vi "AppInit.vi"(10 "path":path, 11 "Changelog":string caption="App Ver") -> (0 "error out":errorcluster)   [LabVIEW 2016]
doc: "Init Host application"
uses:
  Tools/Windows/Windows.ExitAction.ctl
  Tools/EventLog/EventLog.Buffer.Action.ctl
  Tools/Translator/Translator.Message.ctl
  Tools/EventLog/EventLog.New(single).vi
  Global/ApplicationGlobal.vi
  Tools/Config/Config.Global.vi
  Tools/EventLog/EventLog.File.ReadWrite.vi
panel:
  out "idx":i32
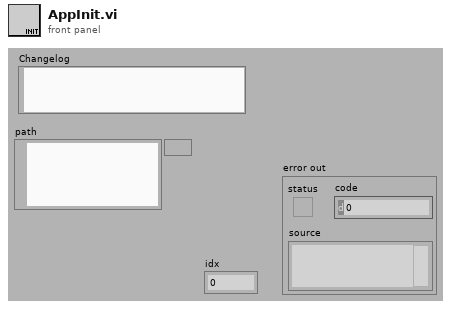
[diagram p1: front panel]
types:
  T1 = typedef "Windows.ExitAction.ctl" = enum16{"Log off from PC", "Shut Down PC", "Reboot PC", "Close Program"}
  T2 = typedef "EventLog.Buffer.Action.ctl" = enum16{"init", "re-init", "clear", "set translator", "translate", "add", "get"}
  T3 = typedef "Translator.Message.ctl" = enum16{"-", "Event confirmed", "Log out", "Log in", "Shutdown", "Cancel", "Start", "Continue", "Stop", "On", "Off", "OK", "NOK", "NOK %s", "This", "Prev", "Home", "Work", "In progress...", "Missing", "Empty", "Hardware failure", "Initial", "Error %d >> %s", "Error %d >> %s >> %s", "Starting %s", "Quitting %s", "Configured", "Initializing", "Quitting", "Loading", "Running %s", "Stopped", "Summary", "Do you want to continue?", "Do you want to exit?", "Log out?", "System", "All", "IDLE", "Translating...%s", "Not found", "Alarm %s", "Run", "Skip", "Abort", "Repeat", "Please wait...", "Database disconnected", "Login to database successful", "Login to database failed: %d; %s", "Get process step data for %s", "Changeover off", "Changeover into %s", "Product %s | %s found in cache with status %d at previous station", "Product %s | %s found in database with status %d at previous station", "Product %s | %s not found in cache at previous station", "Product %s | %s not found in database at previous station", "Product %s | %s found in cache with status %d at this station (%d repetion)", "Product %s | %s found in database with status %d at this station (%d repetition)", "Product %s | %s not found in cache at this station", "Product %s | %s not found in database at this station", "Product %s | %s found in cache for component %s | %s", "Product %s | %s found in database for component %s | %s", "Product not found in cache for component %s | %s", "Product not found in database for component %s | %s", "Product %s | %s connected with component %s | %s (cache)", "Product %s | %s connected with component %s | %s (database)", "New data for %s | %s (cache)", "New data for %s | %s (database)", "File %s moved (cache)", "File %s deleted (cache)", "Msg %d >> %s", "PLC LifeBit Failure", "Reconnecting DB", "Reconnecting PLC", "Free disk space is below 1GB - contact technician"}
  T4 = enum32{"invalid app kind", "Development System", "Run Time System", "Student Edition", "Embedded LabVIEW", "Evaluation", "Custom"}
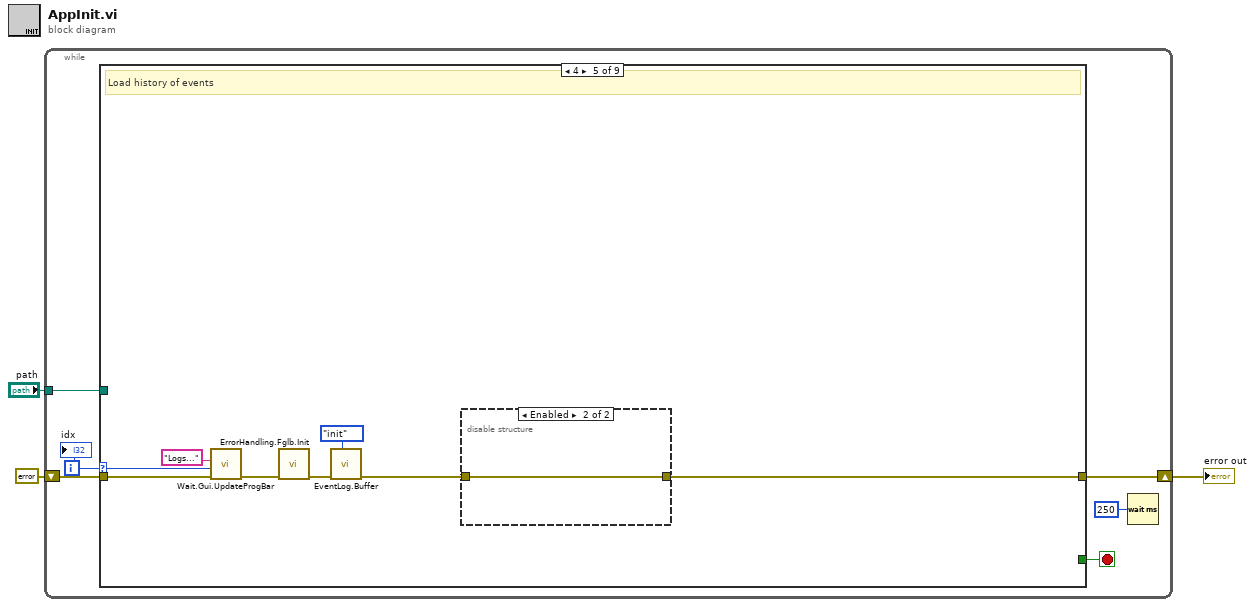
[diagram p0: block diagram]
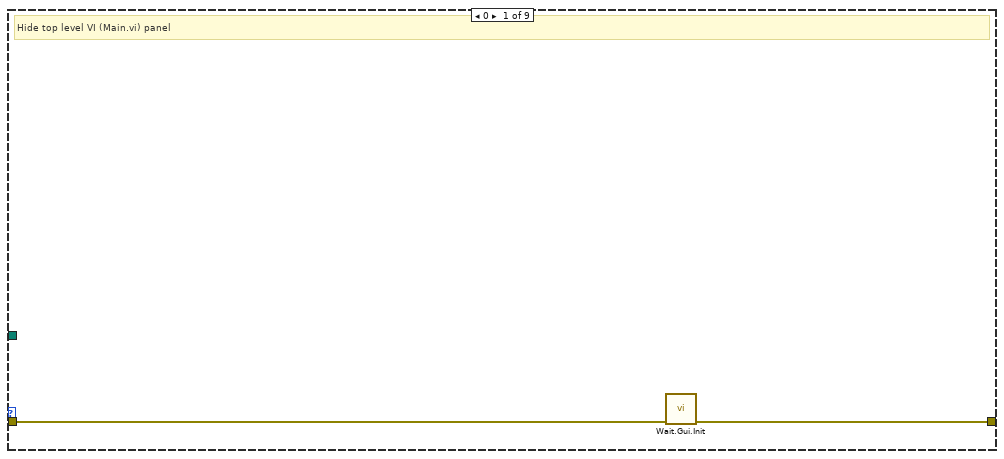
[diagram p2: hidden frame]
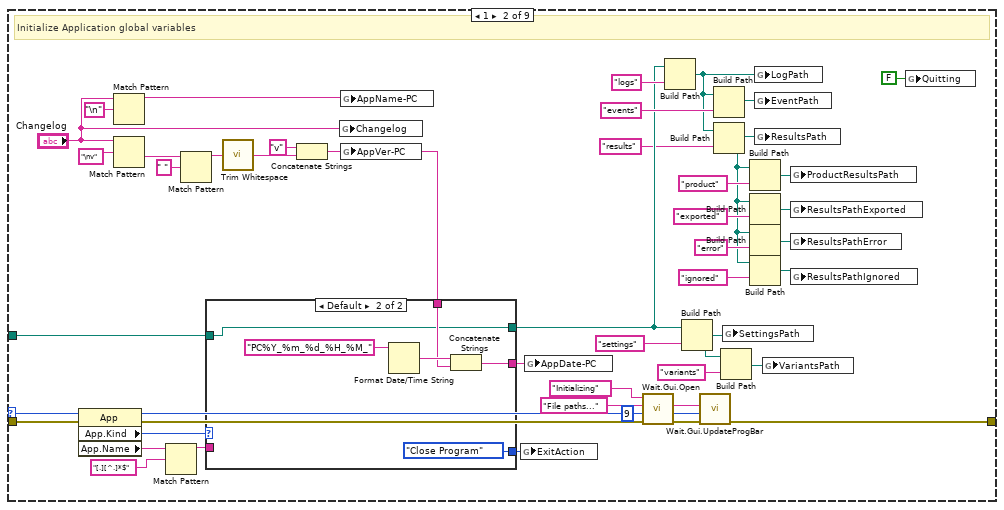
[diagram p3: hidden frame]
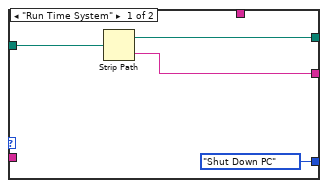
[diagram p4: hidden frame]
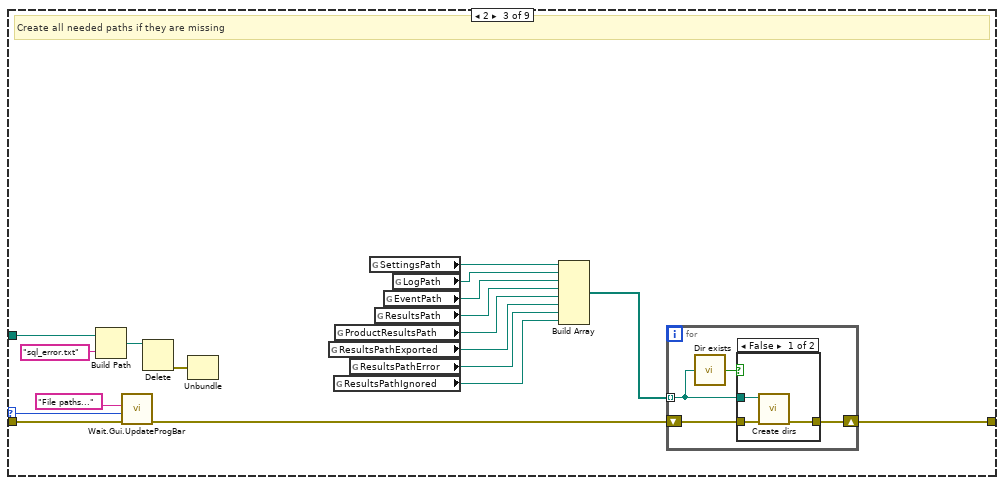
[diagram p5: hidden frame]
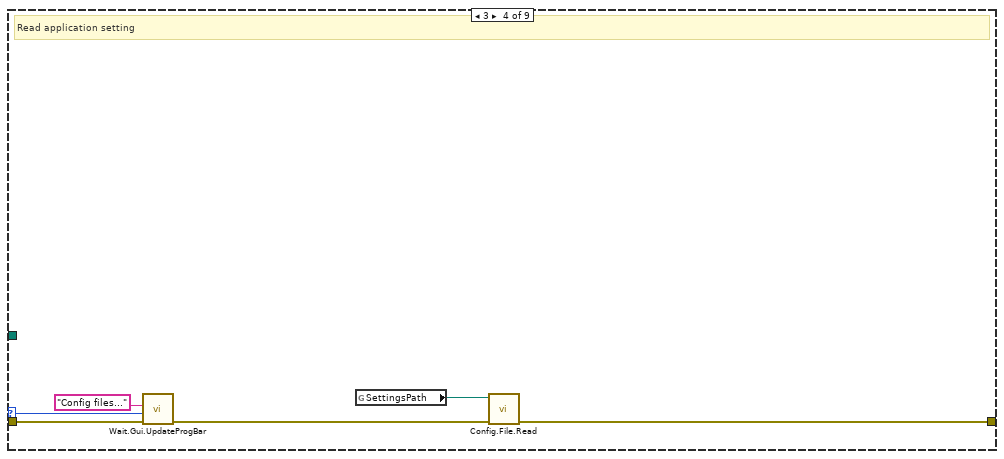
[diagram p7: hidden frame]
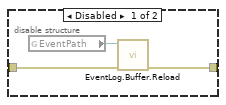
[diagram p8: hidden frame]
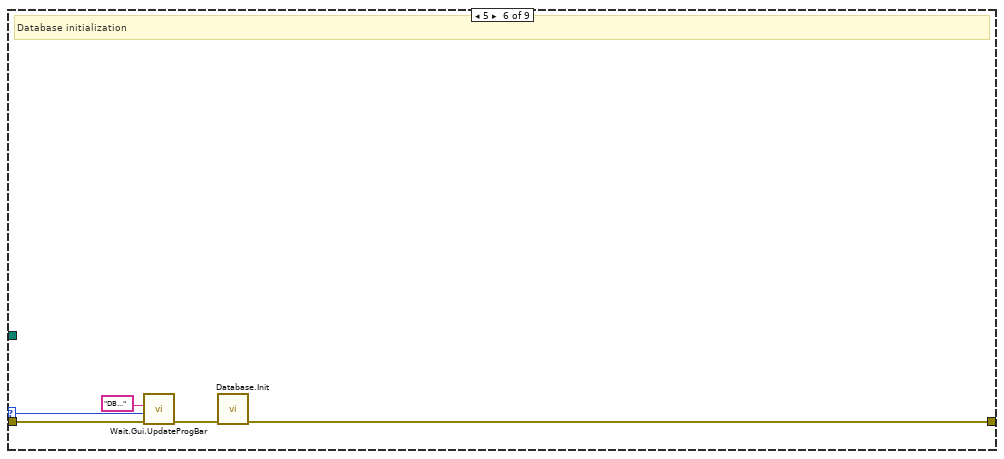
[diagram p9: hidden frame]
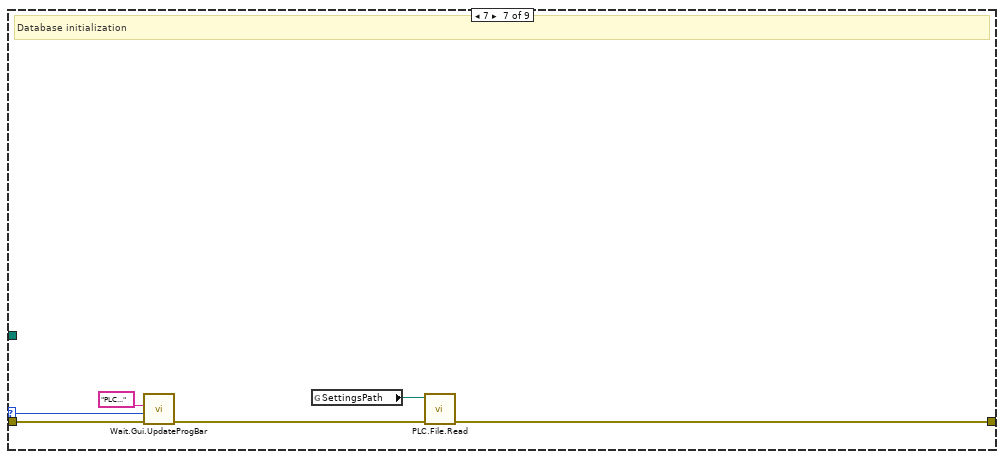
[diagram p10: hidden frame]
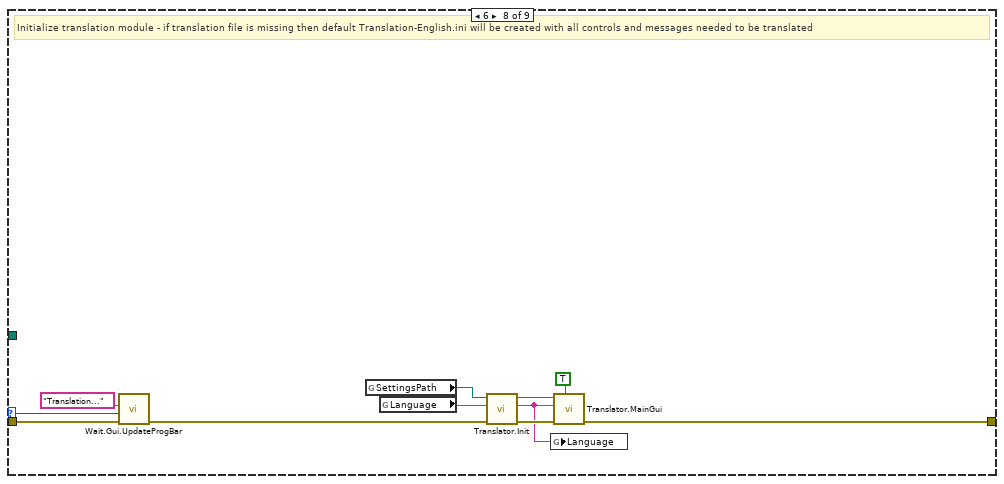
[diagram p11: hidden frame]
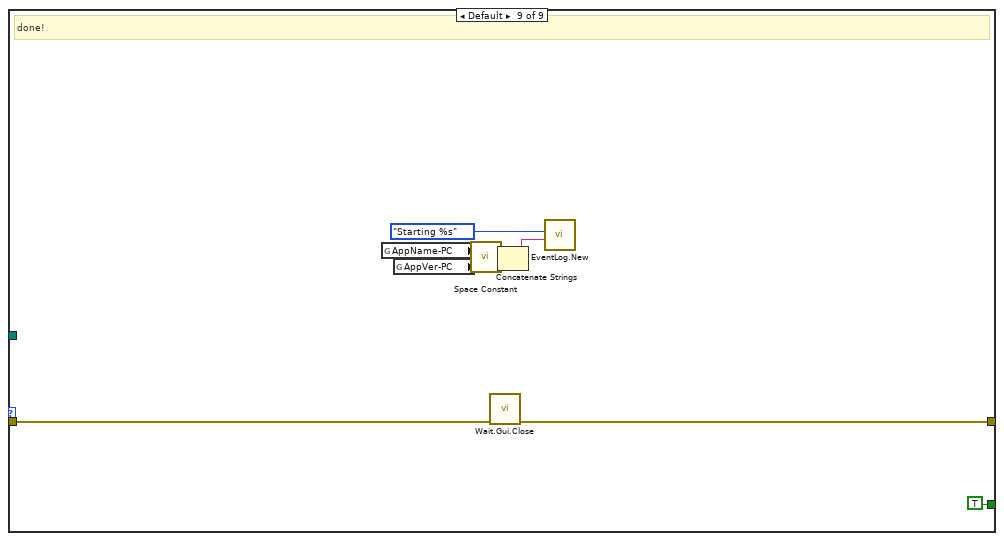
[diagram p12: hidden frame]
diagram:
  n1 = while {
    shift-right: [w7] -> w1
    shift-left: errorcluster {"status"=FALSE, "code"=0, "source"=""} ("error out") -> [w9]
    tunnel: "path" -> [w6]
    i -> [w5]
    stop <- w8 stop-if-true
    n2 = case shown="4" w5 {
      selector: w5 -> [_ w28 w78 w97 w102 w114 w121 w124 _]
      tunnel: w9 -> [w11 w46 w77 w96 w101 w113 w120 w125 w138]
      tunnel: [_ _ _ _ _ _ _ _ TRUE] -> w8
      tunnel: [w10 w29 w81 w93 w99 w115 w117 w123 w137] -> w7
      tunnel: w6 -> [_ w37 w73 _ _ _ _ _ _]
      frame 0 {
        # "Hide top level VI (Main.vi) panel"
        n3 = call "Wait.Gui.Init.vi"("error in (no error)"=w11) -> ("error out"=w10:errorcluster)  [unwired: 10 in]
      }
      frame 1 {
        w32 = "File paths..."
        # "Initialize Application global variables"
        n4 = property class="App"(error in=w46) -> (error out=w30:errorcluster, "App.Kind"=w47:T4, "App.Name"=w40:string)  [unwired: 1 in, 1 out]
        n5 = Match Pattern(string="Changelog", regular expression="\n") -> (before substring=w35:string)  [unwired: 1 in, 3 out]
        n6 = Match Pattern(string="Changelog", regular expression="\nv") -> (after substring=w54:string)  [unwired: 1 in, 3 out]
        n7 = Match Pattern(string=w40, regular expression="[.][^.]*$") -> (before substring=w39:string)  [unwired: 4 out]
        n8 = Match Pattern(string=w54, regular expression=" ") -> (before substring=w51:string)  [unwired: 1 in, 3 out]
        n9 = call <vilib>:"Trim Whitespace.vi"("string"=w51) -> ("trimmed string"=w49:string)  [unwired: 1 in]
        n10 = Concatenate Strings("v" ("string"), w49) -> (w34:string)
        n11 = case shown="Default" w47 {
          tunnel: [w58 w64] -> w43
          tunnel: w34 -> [_ w63]
          tunnel: [w60 w62] -> w27
          tunnel: w39 -> [_ _]
          tunnel: w37 -> [w59 w62]
          tunnel: [Windows.ExitAction."Shut Down PC" ("ExitAction") Windows.ExitAction."Close Program" ("ExitAction")] -> w26
          frame "Run Time System" {
            n12 = Strip Path(path=w59) -> (stripped path=w60:path, name=w58:string)
          }
          frame Default {
            n13 = Format Date/Time String(time format string (%c)="PC%Y_%m_%d_%H_%M_") -> (date/time string=w65:string)  [unwired: 2 in]
            n14 = Concatenate Strings(w65, w63) -> (w64:string)
          }
        }
        n15 = global write "ApplicationGlobal.vi" "Changelog"("Changelog") -> ()
        n16 = global write "ApplicationGlobal.vi" "AppName-PC"(w35) -> ()
        n17 = global write "ApplicationGlobal.vi" "AppVer-PC"(w34) -> ()
        n18 = global write "ApplicationGlobal.vi" "ExitAction"(w26) -> ()
        n19 = global write "ApplicationGlobal.vi" "AppDate-PC"(w43) -> ()
        n20 = call "Wait.Gui.Open.vi"("error in (no error)"=w30, "ProgBarSize (0)"=9 ("ProgBarSize"), "Status (\"\")"=w32, "Msg"="Initializing" ("format string")) -> ("error out"=w33:errorcluster)  [unwired: 7 in]
        n21 = Build Path(base path=w27, name or relative path="logs") -> (appended path=w21:path)
        n22 = Build Path(base path=w27, name or relative path="settings") -> (appended path=w23:path)
        n23 = call "Wait.Gui.UpdateProgBar.vi"("error in (no error)"=w33, "ProgBar (0)"=w28, "status (\"\")"=w32) -> ("error out"=w29:errorcluster)  [unwired: 8 in]
        n24 = Build Path(base path=w21, name or relative path="events") -> (appended path=w42:path)
        n25 = Build Path(base path=w21, name or relative path="results") -> (appended path=w15:path)
        n26 = Build Path(base path=w23, name or relative path="variants") -> (appended path=w22:path)
        n27 = global write "ApplicationGlobal.vi" "SettingsPath"(w23) -> ()
        n28 = Build Path(base path=w15, name or relative path="product") -> (appended path=w19:path)
        n29 = Build Path(base path=w15, name or relative path="exported") -> (appended path=w14:path)
        n30 = Build Path(base path=w15, name or relative path="error") -> (appended path=w13:path)
        n31 = Build Path(base path=w15, name or relative path="ignored") -> (appended path=w12:path)
        n32 = global write "ApplicationGlobal.vi" "LogPath"(w21) -> ()
        n33 = global write "ApplicationGlobal.vi" "EventPath"(w42) -> ()
        n34 = global write "ApplicationGlobal.vi" "ResultsPath"(w15) -> ()
        n35 = global write "ApplicationGlobal.vi" "VariantsPath"(w22) -> ()
        n36 = global write "ApplicationGlobal.vi" "ProductResultsPath"(w19) -> ()
        n37 = global write "ApplicationGlobal.vi" "ResultsPathExported"(w14) -> ()
        n38 = global write "ApplicationGlobal.vi" "ResultsPathError"(w13) -> ()
        n39 = global write "ApplicationGlobal.vi" "ResultsPathIgnored"(w12) -> ()
        n40 = global write "ApplicationGlobal.vi" "Quitting"(FALSE ("Quitting")) -> ()
      }
      frame 2 {
        # "Create all needed paths if they are missing"
        n41 = Build Path(base path=w73, name or relative path="sql_error.txt") -> (appended path=w74:path)
        n42 = call "Wait.Gui.UpdateProgBar.vi"("error in (no error)"=w77, "ProgBar (0)"=w78, "status (\"\")"="File paths...") -> ("error out"=w76:errorcluster)  [unwired: 8 in]
        n43 = Delete(path (use dialog)=w74) -> (error out=w72:errorcluster)  [unwired: 4 in, 2 out]
        n44 = Unbundle(w72) -> ()  [unwired: 3 out]
        n45 = global read "ApplicationGlobal.vi" "ResultsPathExported"() -> (w69:path)
        n46 = global read "ApplicationGlobal.vi" "ResultsPathIgnored"() -> (w67:path)
        n47 = global read "ApplicationGlobal.vi" "ProductResultsPath"() -> (w71:path)
        n48 = global read "ApplicationGlobal.vi" "ResultsPathError"() -> (w68:path)
        n49 = global read "ApplicationGlobal.vi" "SettingsPath"() -> (w84:path)
        n50 = global read "ApplicationGlobal.vi" "ResultsPath"() -> (w70:path)
        n51 = global read "ApplicationGlobal.vi" "EventPath"() -> (w82:path)
        n52 = global read "ApplicationGlobal.vi" "LogPath"() -> (w83:path)
        n53 = Build Array(w84, w83, w82, w70, w71, w69, w68, w67) -> (w80:path[])
        n54 = for {
          tunnel: w80 -> [w86] mode=indexing
          shift-right: [w87] -> w81
          shift-left: w76 -> [w88]
          n55 = call "Dir exists.vi"("dir path"=w86) -> ("exists?"=w85:bool)  [unwired: 4 in]
          n56 = case shown="False" w85 {
            tunnel: w86 -> [w91 _]
            tunnel: w88 -> [w90 w92]
            tunnel: [w89 w92] -> w87
            frame False {
              n57 = call "Create dirs.vi"("error in (no error)"=w90, "deepest dir"=w91) -> ("error"=w89:errorcluster)  [unwired: 9 in]
            }
            frame True {
            }
          }
        }
      }
      frame 3 {
        # "Read application setting"
        n58 = call "Wait.Gui.UpdateProgBar.vi"("error in (no error)"=w96, "ProgBar (0)"=w97, "status (\"\")"="Config files...") -> ("error out"=w94:errorcluster)  [unwired: 8 in]
        n59 = global read "ApplicationGlobal.vi" "SettingsPath"() -> (w95:path)
        n60 = call "Config.File.Read.vi"("error in"=w94, "path"=w95) -> ("error out"=w93:errorcluster)  [unwired: 9 in]
      }
      frame 4 {
        # "Load history of events"
        n61 = call "Wait.Gui.UpdateProgBar.vi"("error in (no error)"=w101, "ProgBar (0)"=w102, "status (\"\")"="Logs...") -> ("error out"=w100:errorcluster)  [unwired: 8 in]
        n62 = call "ErrorHandling.Fglb.Init.vi"("error in (no error)"=w100) -> ("error out"=w104:errorcluster)  [unwired: 10 in]
        n63 = call "EventLog.Buffer.vi"("action (get)"=EventLog.Buffer.Action."init" ("action (read)"), "error in"=w104) -> ("error out"=w105:errorcluster)  [unwired: 6 in, 3 out]
        n64 = disable-structure shown="Enabled" {
          disable-tunnel: [w108 w110] -> w99
          disable-tunnel: w105 -> [w107 w110]
          frame Disabled {
            n65 = global read "ApplicationGlobal.vi" "EventPath"() -> (w109:path)
            n66 = call "EventLog.Buffer.Reload.vi"("error in"=w107, "Path"=w109) -> ("error out"=w108:errorcluster)  [unwired: 9 in]
          }
          frame Enabled {
          }
        }
      }
      frame 5 {
        # "Database initialization"
        n67 = call "Wait.Gui.UpdateProgBar.vi"("error in (no error)"=w113, "ProgBar (0)"=w114, "status (\"\")"="DB...") -> ("error out"=w111:errorcluster)  [unwired: 8 in]
        n68 = call "Database.Init.vi"("error in (no error)"=w111) -> ("error out"=w115:errorcluster)  [unwired: 10 in]
      }
      frame 7 {
        # "Database initialization"
        n69 = call "Wait.Gui.UpdateProgBar.vi"("error in (no error)"=w120, "ProgBar (0)"=w121, "status (\"\")"="PLC...") -> ("error out"=w118:errorcluster)  [unwired: 8 in]
        n70 = global read "ApplicationGlobal.vi" "SettingsPath"() -> (w116:path)
        n71 = call "PLC.File.Read.vi"("error in"=w118, "path"=w116) -> ("error out"=w117:errorcluster)  [unwired: 9 in]
      }
      frame 6 {
        # "Initialize translation module - if translation file is missing then default Translation-English.ini will be created with all controls and messages needed to be translated"
        n72 = call "Wait.Gui.UpdateProgBar.vi"("error in (no error)"=w125, "ProgBar (0)"=w124, "status (\"\")"="Translation...") -> ("error out"=w122:errorcluster)  [unwired: 8 in]
        n73 = global read "ApplicationGlobal.vi" "SettingsPath"() -> (w129:path)
        n74 = global read "Config.Global.vi" "Language"() -> (w130:string)
        n75 = call "Translator.Init.vi"("error in"=w122, "Language in"=w130, "Translation folder"=w129) -> ("error out"=w131:errorcluster, "Language out"=w128:string)  [unwired: 7 in]
        n76 = global write "Config.Global.vi" "Language"(w128) -> ()
        n77 = call "Translator.MainGui.vi"("~init (F)"=TRUE ("init (F)"), "~error in"=w131, "~Language in use"=w128, "~Translation folder"=w129) -> ("~error out"=w123:errorcluster)  [unwired: 4 in, 3 out]
      }
      frame Default {
        # "done!"
        n78 = global read "ApplicationGlobal.vi" "AppName-PC"() -> (w135:string)
        n79 = global read "ApplicationGlobal.vi" "AppVer-PC"() -> (w134:string)
        n80 = call <vilib>:"Space Constant.vi"() -> ("String"=w133:string)
        n81 = call "Wait.Gui.Close.vi"("error in (no error)"=w138) -> ("error out"=w137:errorcluster)  [unwired: 10 in]
        n82 = Concatenate Strings(w135, w133, w134) -> (w132:string)
        n83 = call-poly "EventLog.New.vi"("Arg"=w132, "Message (-)"=Translator.Message."Starting %s") -> ()  [unwired: 8 in, 2 out]
      }
    }
    n84 = Wait (ms)(milliseconds to wait=u32 250) -> ()  [unwired: 1 out]
    "idx" <- w5
  }
  "error out" <- w1
